vi "Get Encoder Value.vi"(1 "Motor Angle":dbl, 2 "Encoder Resolution":i32) -> (0 "Encoder Value":i64)   [LabVIEW 2019]
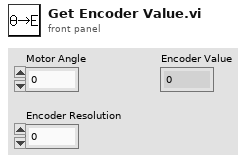
[diagram p1: front panel]
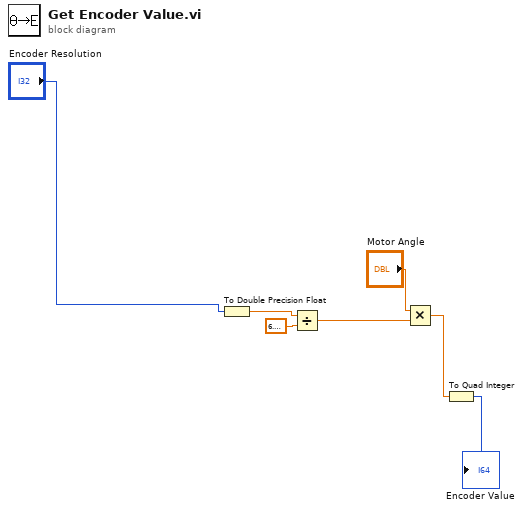
[diagram p0: block diagram]
diagram:
  n1 = To Double Precision Float(number="Encoder Resolution") -> (double precision float=w2:dbl)
  n2 = Divide(x=w2, y=6.283185307179586) -> (x/y=w6:dbl)
  n3 = Multiply(x="Motor Angle", y=w6) -> (x*y=w4:dbl)
  n4 = To Quad Integer(1:w4) -> (0:→"Encoder Value":i64)
